vi "CRYUnflatten Graph Property.vi"(10 "Cluster Name":string, 11 "Flatten Graph Property":string) -> (0 "Error?":bool=TRUE, 2 "Flatten Graph Property Out":string, 3 "Header info":T1={"Data type"="Data            ", "Version"=1, "Dimensions"=0})   [LabVIEW 2013]
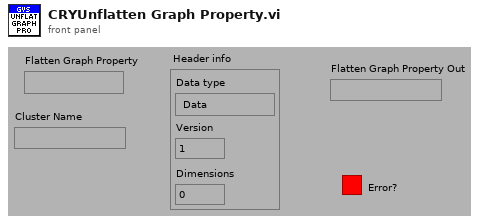
[diagram p1: front panel]
types:
  T1 = cluster{"Data type":string, "Version":u16, "Dimensions":u8}
  T2 = cluster{"unsigned byte array[0]":u8, "unsigned byte array[1]":u8, "unsigned byte array[2]":u8}
  T3 = cluster{"Image Path":string, "Show vertical scroll bar":bool, "Show horizontal scroll bar":bool}
  T4 = cluster{"Show Limits":bool, "Show Yield":bool, "Pass/Fail":bool, "Notation":u16, "Digits":u16, "Precision":u16, "Hide Traling Zeros":bool, "Show vertical scroll bar":bool, "Show horizontal scroll bar":bool, "True":string, "False":string, "Font Size":u16, "Overall/Optional":u16}
  T5 = cluster{"Show Limits":bool, "Show Yield":bool, "Overall Pass/Fail":bool, "Notation":u16, "Digits":u16, "Precision":u16, "Hide Traling Zeros":bool}
  T6 = cluster{"Show Limits":bool, "Show Yield":bool, "Overall Pass/Fail":bool, "Notation":u16, "Digits":u16, "Precision":u16, "Hide Traling Zeros":bool, "Show vertical scroll bar":bool, "Show horizontal scroll bar":bool}
  T7 = cluster{"Show Limits":bool, "Show Yield":bool, "Overall Pass/Fail":bool, "Notation":u16, "Digits":u16, "Precision":u16, "Hide Traling Zeros":bool, "Show vertical scroll bar":bool, "Show horizontal scroll bar":bool, "True":string, "False":string, "Font Size":u16}
  T8 = cluster{"Reset All Columns":bool, "Transpose":bool, "Display Units":bool, "Notation":u16, "Digits":u16, "Precision":u16, "Hide Traling Zeros":bool, "Column Width":u16, "Row Header Width":u16, "Show vertical scroll bar":bool, "Show horizontal scroll bar":bool}
  T9 = cluster{"Reset All Columns":bool, "Transpose":bool, "Display Units":bool, "Notation":u16, "Digits":u16, "Precision":u16, "Hide Traling Zeros":bool, "Column Width":u16, "Row Header Width":u16}
  T10 = cluster{"Time Steps":i32, "Frequency Bins":i32, "Type":u32, "Length":i32, "Map Type":enum16{"fire", "rainbow", "grey", "inverse grey", "ice", "original"}}
  T11 = cluster{"polar attributes":cluster{"maximum":dbl, "minimum":dbl, "clip to min":bool, "log":bool, "grid color":u32, "plot color":u32, "fmt and prec":cluster{"format":enum8{"Decimal", "Scientific", "Engineering", "Binary", "Octal", "Hex"}, "precision":u8}, "visible section":u16}, "Auto/Manual":u16, "Zero Adjust (deg)":i32, "Angle Increment (deg)":i32, "Mirror":bool, "Auto Increment":bool, "Total Rotatin (deg)":i32, "Discrete/Rannge":u16, "Show Name":bool, "CurValues":dbl[], "CurIndex":u16, "CurColors":u32[], "CurColors_Range":u32[], "CurValues_Range":dbl[], "Pen":cluster{"Width":u16, "Style":enum32{"Solid", "Dash", "Dot", "DashDot", "DashDotDot"}}, "BackgroundColor":u32}
  T12 = cluster{"polar attributes":cluster{"maximum":dbl, "minimum":dbl, "clip to min":bool, "log":bool, "grid color":u32, "plot color":u32, "fmt and prec":cluster{"format":enum8{"Decimal", "Scientific", "Engineering", "Binary", "Octal", "Hex"}, "precision":u8}, "visible section":u16}, "Auto/Manual":u16, "Zero Adjust (deg)":i32, "Angle Increment (deg)":i32, "Mirror":bool, "Auto Increment":bool, "Total Rotatin (deg)":i32, "Discrete/Rannge":u16, "Show Name":bool, "CurValues":dbl[], "CurIndex":u16, "CurColors":u32[], "CurColors_Range":u32[], "CurValues_Range":dbl[], "Pen":cluster{"Width":u16, "Style":enum32{"Solid", "Dash", "Dot", "DashDot", "DashDotDot"}}}
  T13 = cluster{"maximum":dbl, "minimum":dbl, "clip to min":bool, "log":bool, "grid color":u32, "plot color":u32, "fmt and prec":cluster{"format":enum8{"Decimal", "Scientific", "Engineering", "Binary", "Octal", "Hex"}, "precision":u8}, "visible section":u16}
  T14 = cluster{"Width":u16, "Style":enum32{"Solid", "Dash", "Dot", "DashDot", "DashDotDot"}}
  T15 = cluster{"Size":u32, "Bold":bool, "Italic":bool, "Underline":bool, "Strikethrough":bool, "Color":u32, "Font":string, "String":string, "Show vertical scroll bar":bool, "Show horizontal scroll bar":bool}
  T16 = cluster{"Size":u32, "Bold":bool, "Italic":bool, "Underline":bool, "Strikethrough":bool, "Color":u32, "Font":string, "String":string}
  T17 = cluster{"substring":string, u16, "unsigned byte array[2]":u8}
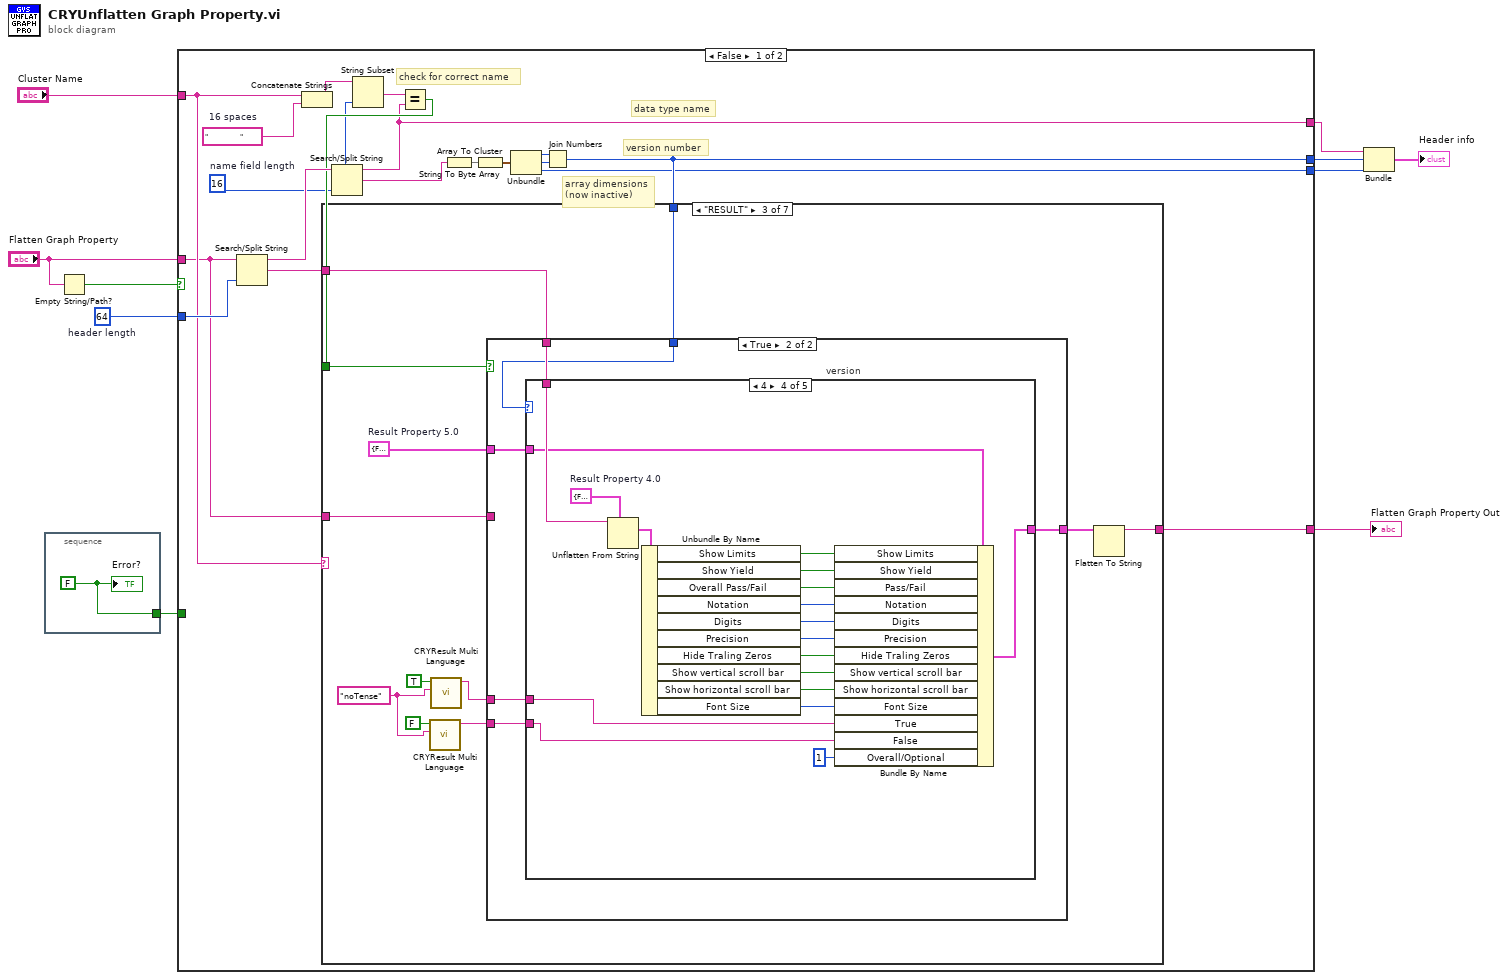
[diagram p0: block diagram]
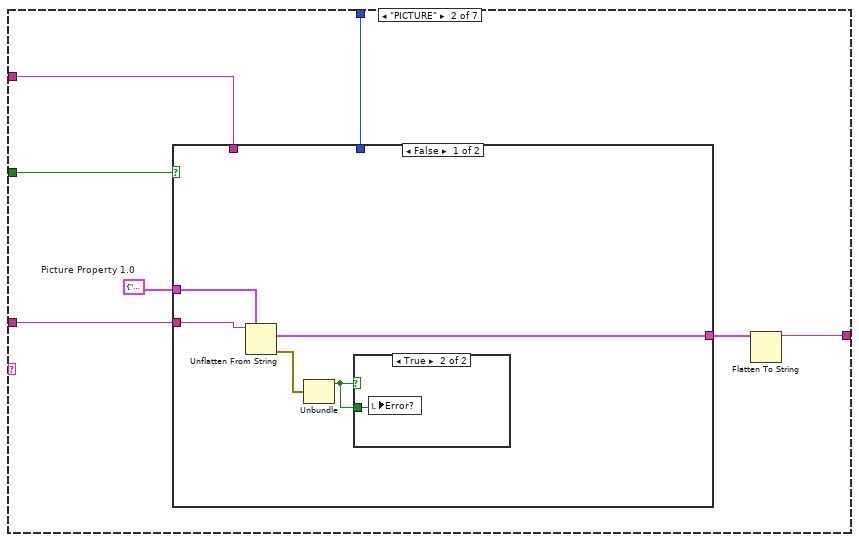
[diagram p3: hidden frame]
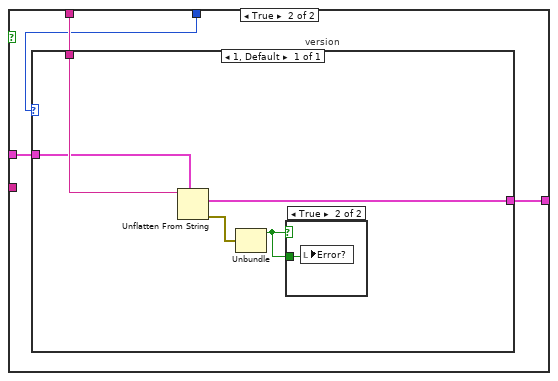
[diagram p5: hidden frame]
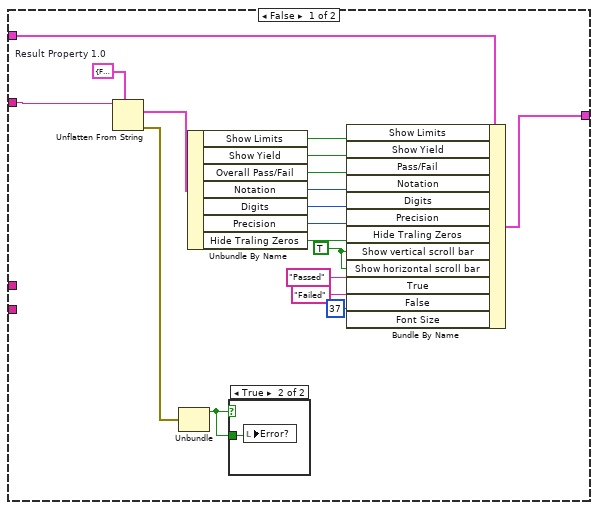
[diagram p7: hidden frame]
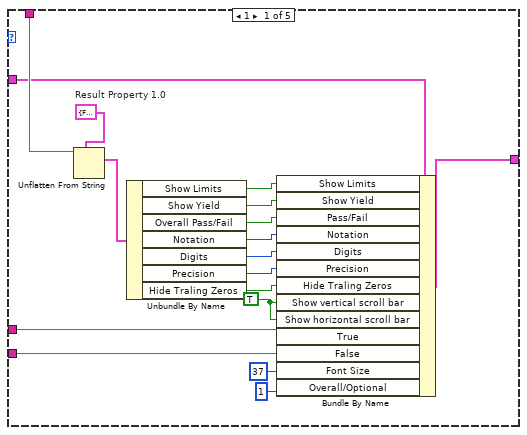
[diagram p9: hidden frame]
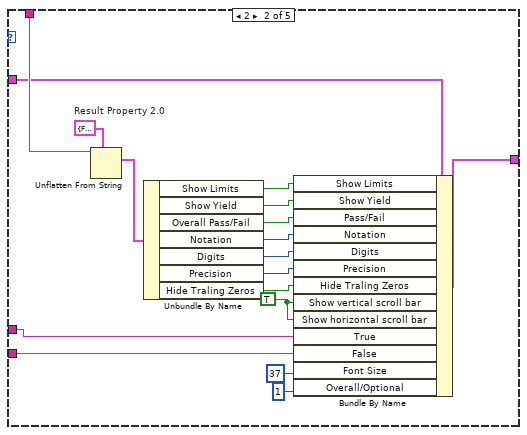
[diagram p10: hidden frame]
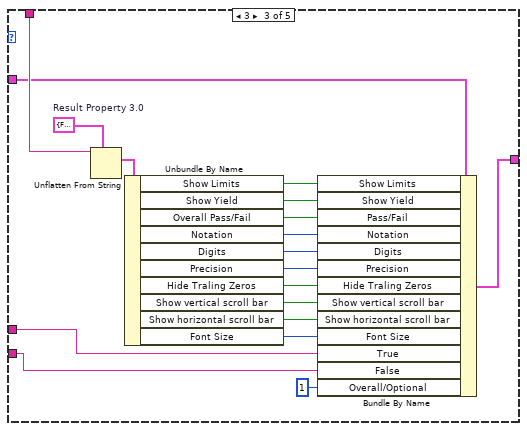
[diagram p11: hidden frame]
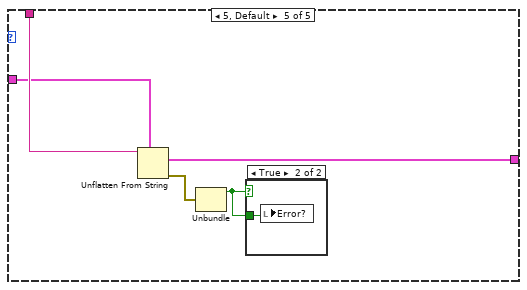
[diagram p12: hidden frame]
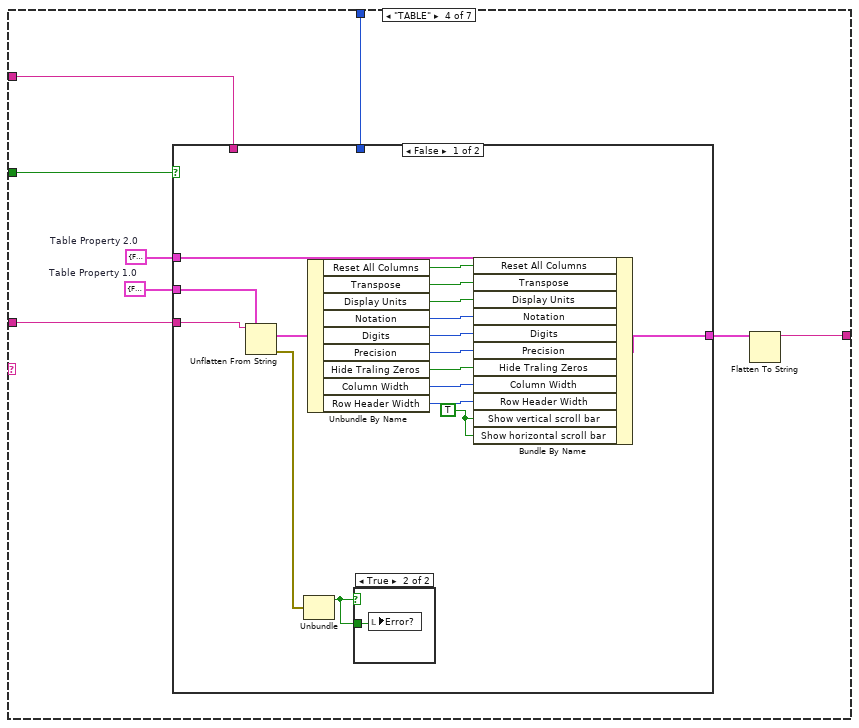
[diagram p14: hidden frame]
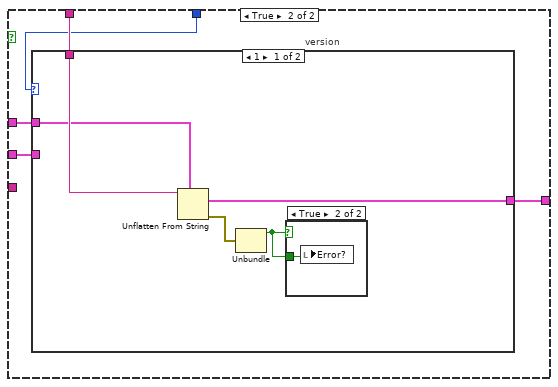
[diagram p16: hidden frame]
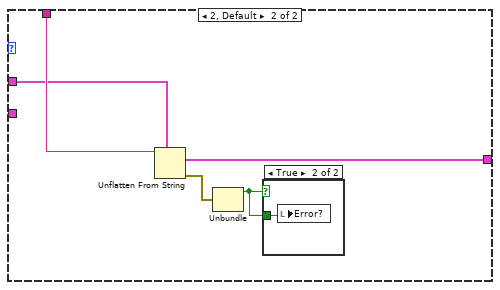
[diagram p18: hidden frame]
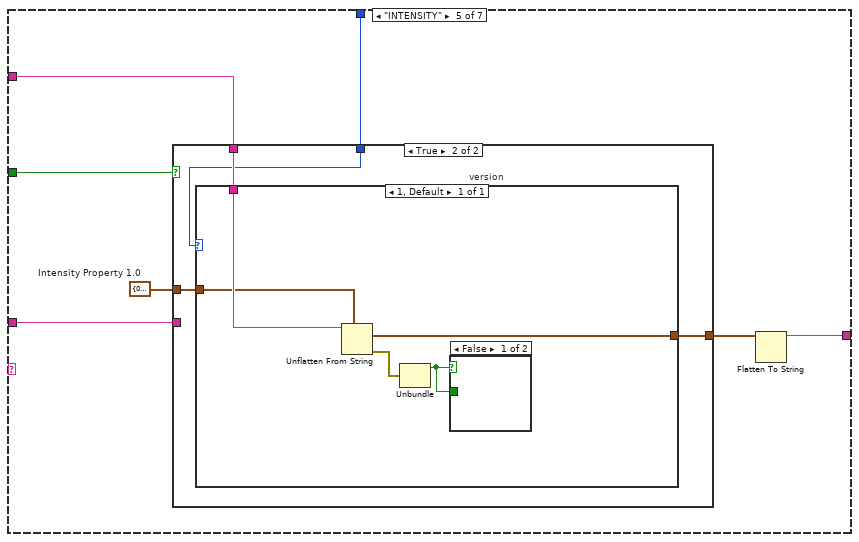
[diagram p20: hidden frame]
diagram:
  w8 = 64  # header length
  n1 = stacked-sequence {
    tunnel: [w11] -> w3
    frame #0 {
      w11 = FALSE
      "Error?" <- w11
    }
  }
  n2 = Empty String/Path?(string/path="Flatten Graph Property") -> (empty?=w9:bool)
  n3 = case shown="False" w9 {
    tunnel: "Flatten Graph Property" -> [w12 _]
    tunnel: w8 -> [w25 _]
    tunnel: [w22 u16 0] -> w6
    tunnel: [w15 u8 0] -> w7
    tunnel: [w16 "(no data input)" ("substring")] -> w5
    tunnel: w3 -> [_ _]
    tunnel: "Cluster Name" -> [w14 _]
    tunnel: [w13 "" ("data string")] -> w1
    frame False {
      w20 = "                "  # 16 spaces
      w18 = 16  # name field length
      # "check for correct name"
      # "array dimensions\n(now inactive)"
      # "version number"
      # "data type name"
      n4 = Search/Split String(string=w12, offset (0)=w25) -> (substring before match=w24:string, match + rest of string=w26:string)  [unwired: 2 out]
      n5 = Concatenate Strings(w14, w20) -> (w19:string)
      n6 = Search/Split String(string=w24, offset (0)=w18) -> (substring before match=w16:string, match + rest of string=w21:string)  [unwired: 2 out]
      n7 = String Subset(string=w19, length (rest)=w18) -> (substring=w17:string)  [unwired: 1 out]
      n8 = Equal?(x=w17, y=w16) -> (x = y?=w23:bool)
      n9 = String To Byte Array(string=w21) -> (unsigned byte array=w30:u8[])
      n10 = Array To Cluster(array=w30) -> (cluster=w29:T2)
      n11 = Unbundle(w29) -> ("unsigned byte array[0]"=w28:u8, "unsigned byte array[1]"=w27:u8, "unsigned byte array[2]"=w15:u8)
      n12 = Join Numbers(hi=w28, lo=w27) -> ((hi.lo)=w22:u16)
      n13 = case shown="\"RESULT\"" w14 {
        tunnel: w26 -> [_ w38 w66 w175 w217 w242 w322]
        tunnel: w23 -> [_ w37 w65 w174 w216 w241 w321]
        tunnel: w22 -> [_ w36 w64 w173 w215 w240 w320]
        tunnel: [w31 w33 w62 w169 w212 w237 w317] -> w13
        tunnel: w12 -> [w31 w32 w61 w168 w211 w236 w316]
        frame Default {
        }
        frame "PICTURE" {
          w35 = T3 {"Image Path"="", "Show vertical scroll bar"=FALSE, "Show horizontal scroll bar"=FALSE}  # Picture Property 1.0
          n14 = case shown="False" w37 {
            tunnel: w38 -> [_ w48]
            tunnel: w36 -> [_ w47]
            tunnel: w35 -> [w41 w46]
            tunnel: [w40 w45] -> w34
            tunnel: w32 -> [w39 _]
            frame False {
              n15 = Unflatten From String(type=w41, binary string=w39) -> (value=w40:T3, error out=w42:errorcluster)  [unwired: 1 in, 3 out]
              n16 = Unbundle(w42) -> ("status"=w43:bool)  [unwired: 2 out]
              n17 = case shown="True" w43 {
                tunnel: w43 -> [_ w44]
                frame False {
                }
                frame True {
                  n18 = local write "Error?"(w44) -> ()
                }
              }
            }
            frame True {
              n19 = case "version" shown="1, Default" w47 {
                tunnel: w48 -> [w53]
                tunnel: w46 -> [w50]
                tunnel: [w49] -> w45
                frame 1, Default {
                  n20 = Unflatten From String(type=w50, binary string=w53) -> (value=w49:T3, error out=w51:errorcluster)  [unwired: 1 in, 3 out]
                  n21 = Unbundle(w51) -> ("status"=w52:bool)  [unwired: 2 out]
                  n22 = case shown="True" w52 {
                    tunnel: w52 -> [_ w54]
                    frame False {
                    }
                    frame True {
                      n23 = local write "Error?"(w54) -> ()
                    }
                  }
                }
              }
            }
          }
          n24 = Flatten To String(anything=w34) -> (data string=w33:string)  [unwired: 3 in, 2 out]
        }
        frame "RESULT" {
          w55 = "noTense" ("sOption")
          w56 = T4 {"Show Limits"=FALSE, "Show Yield"=FALSE, "Pass/Fail"=FALSE, "Notation"=0, "Digits"=0, "Precision"=0, "Hide Traling Zeros"=FALSE, "Show vertical scroll bar"=FALSE, "Show horizontal scroll bar"=FALSE, "True"="NO ELECTRICAL SIGNAL DETECTED!\nCheck wiring and connections.", "False"="NO ELECTRICAL SIGNAL DETECTED!\nCheck wiring and connections.", "Font Size"=0, "Overall/Optional"=0}  # Result Property 5.0
          n25 = call "CRYResult Multi Language.vi"("sOption"=w55, "Verdict"=FALSE) -> ("ASCII out"=w57:string)  [unwired: 9 in]
          n26 = call "CRYResult Multi Language.vi"("sOption"=w55, "Verdict"=TRUE) -> ("ASCII out"=w58:string)  [unwired: 9 in]
          n27 = case shown="True" w65 {
            tunnel: w66 -> [_ w91]
            tunnel: w64 -> [_ w90]
            tunnel: [w71 w89] -> w63
            tunnel: w61 -> [w82 _]
            tunnel: w56 -> [w81 w88]
            tunnel: w58 -> [_ w87]
            tunnel: w57 -> [_ w86]
            frame False {
              w70 = T5 {"Show Limits"=FALSE, "Show Yield"=FALSE, "Overall Pass/Fail"=FALSE, "Notation"=0, "Digits"=0, "Precision"=0, "Hide Traling Zeros"=FALSE}  # Result Property 1.0
              w73 = TRUE ("Show vertical scroll bar")
              n28 = Unflatten From String(type=w70, binary string=w82) -> (value=w72:T5, error out=w83:errorcluster)  [unwired: 1 in, 3 out]
              n29 = Unbundle(w83) -> ("status"=w84:bool)  [unwired: 2 out]
              n30 = Unbundle By Name(w72) -> ("Show Limits"=w80:bool, "Show Yield"=w79:bool, "Overall Pass/Fail"=w78:bool, "Notation"=w77:u16, "Digits"=w76:u16, "Precision"=w75:u16, "Hide Traling Zeros"=w74:bool)
              n31 = case shown="True" w84 {
                tunnel: w84 -> [_ w85]
                frame False {
                }
                frame True {
                  n32 = local write "Error?"(w85) -> ()
                }
              }
              n33 = Bundle By Name(cluster=w81, "Show Limits"=w80, "Show Yield"=w79, "Pass/Fail"=w78, "Notation"=w77, "Digits"=w76, "Precision"=w75, "Hide Traling Zeros"=w74, "Show vertical scroll bar"=w73, "Show horizontal scroll bar"=w73, "True"="Passed", "False"="Failed", "Font Size"=u16 37) -> (w71:T4)
            }
            frame True {
              n34 = case "version" shown="4" w90 {
                tunnel: w91 -> [w108 w125 w143 w161 w166]
                tunnel: [w97 w114 w133 w151 w163] -> w89
                tunnel: w88 -> [w107 w124 w142 w160 w162]
                tunnel: w87 -> [w94 w110 w128 w147 _]
                tunnel: w86 -> [w93 w111 w127 w146 _]
                frame 1 {
                  w96 = T5 {"Show Limits"=FALSE, "Show Yield"=FALSE, "Overall Pass/Fail"=FALSE, "Notation"=0, "Digits"=0, "Precision"=0, "Hide Traling Zeros"=FALSE}  # Result Property 1.0
                  w99 = TRUE ("Show vertical scroll bar")
                  n35 = Unflatten From String(type=w96, binary string=w108) -> (value=w98:T5)  [unwired: 1 in, 4 out]
                  n36 = Unbundle By Name(w98) -> ("Show Limits"=w106:bool, "Show Yield"=w105:bool, "Overall Pass/Fail"=w104:bool, "Notation"=w103:u16, "Digits"=w102:u16, "Precision"=w101:u16, "Hide Traling Zeros"=w100:bool)
                  n37 = Bundle By Name(cluster=w107, "Show Limits"=w106, "Show Yield"=w105, "Pass/Fail"=w104, "Notation"=w103, "Digits"=w102, "Precision"=w101, "Hide Traling Zeros"=w100, "Show vertical scroll bar"=w99, "Show horizontal scroll bar"=w99, "True"=w94, "False"=w93, "Font Size"=u16 37, "Overall/Optional"=u16 1) -> (w97:T4)
                }
                frame 2 {
                  w113 = T6 {"Show Limits"=FALSE, "Show Yield"=FALSE, "Overall Pass/Fail"=FALSE, "Notation"=0, "Digits"=0, "Precision"=0, "Hide Traling Zeros"=FALSE, "Show vertical scroll bar"=FALSE, "Show horizontal scroll bar"=FALSE}  # Result Property 2.0
                  w116 = TRUE ("Show vertical scroll bar")
                  n38 = Unflatten From String(type=w113, binary string=w125) -> (value=w115:T6)  [unwired: 1 in, 4 out]
                  n39 = Unbundle By Name(w115) -> ("Show Limits"=w123:bool, "Show Yield"=w122:bool, "Overall Pass/Fail"=w121:bool, "Notation"=w120:u16, "Digits"=w119:u16, "Precision"=w118:u16, "Hide Traling Zeros"=w117:bool)
                  n40 = Bundle By Name(cluster=w124, "Show Limits"=w123, "Show Yield"=w122, "Pass/Fail"=w121, "Notation"=w120, "Digits"=w119, "Precision"=w118, "Hide Traling Zeros"=w117, "Show vertical scroll bar"=w116, "Show horizontal scroll bar"=w116, "True"=w110, "False"=w111, "Font Size"=u16 37, "Overall/Optional"=u16 1) -> (w114:T4)
                }
                frame 3 {
                  w130 = T7 {"Show Limits"=FALSE, "Show Yield"=FALSE, "Overall Pass/Fail"=FALSE, "Notation"=0, "Digits"=0, "Precision"=0, "Hide Traling Zeros"=FALSE, "Show vertical scroll bar"=FALSE, "Show horizontal scroll bar"=FALSE, "True"="", "False"="", "Font Size"=2}  # Result Property 3.0
                  n41 = Unflatten From String(type=w130, binary string=w143) -> (value=w134:T7)  [unwired: 1 in, 4 out]
                  n42 = Unbundle By Name(w134) -> ("Show Limits"=w141:bool, "Show Yield"=w140:bool, "Overall Pass/Fail"=w139:bool, "Notation"=w138:u16, "Digits"=w137:u16, "Precision"=w136:u16, "Hide Traling Zeros"=w135:bool, "Show vertical scroll bar"=w132:bool, "Show horizontal scroll bar"=w131:bool, "Font Size"=w129:u16)
                  n43 = Bundle By Name(cluster=w142, "Show Limits"=w141, "Show Yield"=w140, "Pass/Fail"=w139, "Notation"=w138, "Digits"=w137, "Precision"=w136, "Hide Traling Zeros"=w135, "Show vertical scroll bar"=w132, "Show horizontal scroll bar"=w131, "Font Size"=w129, "True"=w128, "False"=w127, "Overall/Optional"=u16 1) -> (w133:T4)
                }
                frame 4 {
                  w145 = T7 {"Show Limits"=FALSE, "Show Yield"=FALSE, "Overall Pass/Fail"=FALSE, "Notation"=0, "Digits"=0, "Precision"=0, "Hide Traling Zeros"=FALSE, "Show vertical scroll bar"=FALSE, "Show horizontal scroll bar"=FALSE, "True"="", "False"="", "Font Size"=2}  # Result Property 4.0
                  n44 = Unflatten From String(type=w145, binary string=w161) -> (value=w152:T7)  [unwired: 1 in, 4 out]
                  n45 = Unbundle By Name(w152) -> ("Show Limits"=w159:bool, "Show Yield"=w158:bool, "Overall Pass/Fail"=w157:bool, "Notation"=w156:u16, "Digits"=w155:u16, "Precision"=w154:u16, "Hide Traling Zeros"=w153:bool, "Show vertical scroll bar"=w150:bool, "Show horizontal scroll bar"=w149:bool, "Font Size"=w148:u16)
                  n46 = Bundle By Name(cluster=w160, "Show Limits"=w159, "Show Yield"=w158, "Pass/Fail"=w157, "Notation"=w156, "Digits"=w155, "Precision"=w154, "Hide Traling Zeros"=w153, "Show vertical scroll bar"=w150, "Show horizontal scroll bar"=w149, "Font Size"=w148, "True"=w147, "False"=w146, "Overall/Optional"=u16 1) -> (w151:T4)
                }
                frame 5, Default {
                  n47 = Unflatten From String(type=w162, binary string=w166) -> (value=w163:T4, error out=w164:errorcluster)  [unwired: 1 in, 3 out]
                  n48 = Unbundle(w164) -> ("status"=w165:bool)  [unwired: 2 out]
                  n49 = case shown="True" w165 {
                    tunnel: w165 -> [_ w167]
                    frame False {
                    }
                    frame True {
                      n50 = local write "Error?"(w167) -> ()
                    }
                  }
                }
              }
            }
          }
          n51 = Flatten To String(anything=w63) -> (data string=w62:string)  [unwired: 3 in, 2 out]
        }
        frame "TABLE" {
          w171 = T8 {"Reset All Columns"=FALSE, "Transpose"=FALSE, "Display Units"=FALSE, "Notation"=0, "Digits"=0, "Precision"=0, "Hide Traling Zeros"=FALSE, "Column Width"=0, "Row Header Width"=0, "Show vertical scroll bar"=FALSE, "Show horizontal scroll bar"=FALSE}  # Table Property 2.0
          w172 = T9 {"Reset All Columns"=FALSE, "Transpose"=FALSE, "Display Units"=FALSE, "Notation"=0, "Digits"=0, "Precision"=0, "Hide Traling Zeros"=FALSE, "Column Width"=0, "Row Header Width"=0}  # Table Property 1.0
          n52 = case shown="False" w174 {
            tunnel: w175 -> [_ w198]
            tunnel: w173 -> [_ w197]
            tunnel: w172 -> [w190 w196]
            tunnel: [w187 w195] -> w170
            tunnel: w171 -> [w188 w194]
            tunnel: w168 -> [w176 _]
            frame False {
              w177 = TRUE ("Show vertical scroll bar")
              n53 = Unflatten From String(type=w190, binary string=w176) -> (value=w189:T9, error out=w191:errorcluster)  [unwired: 1 in, 3 out]
              n54 = Unbundle(w191) -> ("status"=w192:bool)  [unwired: 2 out]
              n55 = Unbundle By Name(w189) -> ("Reset All Columns"=w186:bool, "Transpose"=w185:bool, "Display Units"=w184:bool, "Notation"=w183:u16, "Digits"=w182:u16, "Precision"=w181:u16, "Hide Traling Zeros"=w180:bool, "Column Width"=w179:u16, "Row Header Width"=w178:u16)
              n56 = case shown="True" w192 {
                tunnel: w192 -> [_ w193]
                frame False {
                }
                frame True {
                  n57 = local write "Error?"(w193) -> ()
                }
              }
              n58 = Bundle By Name(cluster=w188, "Reset All Columns"=w186, "Transpose"=w185, "Display Units"=w184, "Notation"=w183, "Digits"=w182, "Precision"=w181, "Hide Traling Zeros"=w180, "Column Width"=w179, "Row Header Width"=w178, "Show vertical scroll bar"=w177, "Show horizontal scroll bar"=w177) -> (w187:T8)
            }
            frame True {
              n59 = case "version" shown="1" w197 {
                tunnel: w198 -> [w203 w209]
                tunnel: w196 -> [_ _]
                tunnel: [w200 w206] -> w195
                tunnel: w194 -> [w199 w205]
                frame 1 {
                  n60 = Unflatten From String(type=w199, binary string=w203) -> (value=w200:T8, error out=w201:errorcluster)  [unwired: 1 in, 3 out]
                  n61 = Unbundle(w201) -> ("status"=w202:bool)  [unwired: 2 out]
                  n62 = case shown="True" w202 {
                    tunnel: w202 -> [_ w204]
                    frame False {
                    }
                    frame True {
                      n63 = local write "Error?"(w204) -> ()
                    }
                  }
                }
                frame 2, Default {
                  n64 = Unflatten From String(type=w205, binary string=w209) -> (value=w206:T8, error out=w207:errorcluster)  [unwired: 1 in, 3 out]
                  n65 = Unbundle(w207) -> ("status"=w208:bool)  [unwired: 2 out]
                  n66 = case shown="True" w208 {
                    tunnel: w208 -> [_ w210]
                    frame False {
                    }
                    frame True {
                      n67 = local write "Error?"(w210) -> ()
                    }
                  }
                }
              }
            }
          }
          n68 = Flatten To String(anything=w170) -> (data string=w169:string)  [unwired: 3 in, 2 out]
        }
        frame "INTENSITY" {
          w214 = T10 {"Time Steps"=0, "Frequency Bins"=0, "Type"=0, "Length"=0, "Map Type"=enum."fire"}  # Intensity Property 1.0
          n69 = case shown="True" w216 {
            tunnel: w217 -> [_ w227]
            tunnel: w215 -> [_ w226]
            tunnel: w214 -> [w220 w225]
            tunnel: [w219 w224] -> w213
            tunnel: w211 -> [w218 _]
            frame False {
              n70 = Unflatten From String(type=w220, binary string=w218) -> (value=w219:T10, error out=w221:errorcluster)  [unwired: 1 in, 3 out]
              n71 = Unbundle(w221) -> ("status"=w222:bool)  [unwired: 2 out]
              n72 = case shown="True" w222 {
                tunnel: w222 -> [_ w223]
                frame False {
                }
                frame True {
                  n73 = local write "Error?"(w223) -> ()
                }
              }
            }
            frame True {
              n74 = case "version" shown="1, Default" w226 {
                tunnel: w227 -> [w232]
                tunnel: w225 -> [w229]
                tunnel: [w228] -> w224
                frame 1, Default {
                  n75 = Unflatten From String(type=w229, binary string=w232) -> (value=w228:T10, error out=w230:errorcluster)  [unwired: 1 in, 3 out]
                  n76 = Unbundle(w230) -> ("status"=w231:bool)  [unwired: 2 out]
                  n77 = case shown="False" w231 {
                    tunnel: w231 -> [_ w233]
                    frame False {
                    }
                    frame True {
                      n78 = local write "Error?"(w233) -> ()
                    }
                  }
                }
              }
            }
          }
          n79 = Flatten To String(anything=w213) -> (data string=w212:string)  [unwired: 3 in, 2 out]
        }
        frame "POLAR" {
          w234 = T11 {"polar attributes"={"maximum"=2.0, "minimum"=0.0, "clip to min"=FALSE, "log"=FALSE, "grid color"=3381657, "plot color"=16711680, "fmt and prec"={"format"=enum."Decimal", "precision"=2}, "visible section"=4}, "Auto/Manual"=0, "Zero Adjust (deg)"=0, "Angle Increment (deg)"=0, "Mirror"=FALSE, "Auto Increment"=FALSE, "Total Rotatin (deg)"=0, "Discrete/Rannge"=0, "Show Name"=FALSE, "CurValues"=[], "CurIndex"=0, "CurColors"=[], "CurColors_Range"=[], "CurValues_Range"=[], "Pen"={"Width"=1, "Style"=enum."Solid"}, "BackgroundColor"=0}  # Polar Property 3.0
          w235 = T12 {"polar attributes"={"maximum"=2.0, "minimum"=0.0, "clip to min"=FALSE, "log"=FALSE, "grid color"=3381657, "plot color"=16711680, "fmt and prec"={"format"=enum."Decimal", "precision"=2}, "visible section"=4}, "Auto/Manual"=0, "Zero Adjust (deg)"=0, "Angle Increment (deg)"=0, "Mirror"=FALSE, "Auto Increment"=FALSE, "Total Rotatin (deg)"=0, "Discrete/Rannge"=0, "Show Name"=FALSE, "CurValues"=[], "CurIndex"=0, "CurColors"=[], "CurColors_Range"=[], "CurValues_Range"=[], "Pen"={"Width"=1, "Style"=enum."Solid"}}  # Polar Property 2.0
          w239 = T12 {"polar attributes"={"maximum"=2.0, "minimum"=0.0, "clip to min"=FALSE, "log"=FALSE, "grid color"=3381657, "plot color"=16711680, "fmt and prec"={"format"=enum."Decimal", "precision"=2}, "visible section"=4}, "Auto/Manual"=0, "Zero Adjust (deg)"=0, "Angle Increment (deg)"=0, "Mirror"=FALSE, "Auto Increment"=FALSE, "Total Rotatin (deg)"=0, "Discrete/Rannge"=0, "Show Name"=FALSE, "CurValues"=[], "CurIndex"=0, "CurColors"=[], "CurColors_Range"=[], "CurValues_Range"=[], "Pen"={"Width"=1, "Style"=enum."Solid"}}  # Polar Property 1.0
          n80 = case shown="True" w241 {
            tunnel: w242 -> [_ w269]
            tunnel: w240 -> [_ w268]
            tunnel: w239 -> [w262 w267]
            tunnel: [w245 w266] -> w238
            tunnel: w236 -> [w263 _]
            tunnel: w235 -> [_ w265]
            tunnel: w234 -> [w244 w264]
            frame False {
              n81 = Unflatten From String(type=w262, binary string=w263) -> (value=w246:T12)  [unwired: 1 in, 4 out]
              n82 = Unbundle By Name(w246) -> ("polar attributes"=w261:T13, "Auto/Manual"=w260:u16, "Zero Adjust (deg)"=w259:i32, "Angle Increment (deg)"=w258:i32, "Mirror"=w257:bool, "Auto Increment"=w256:bool, "Total Rotatin (deg)"=w255:i32, "Discrete/Rannge"=w254:u16, "Show Name"=w253:bool, "CurValues"=w252:dbl[], "CurIndex"=w251:u16, "CurColors"=w250:u32[], "CurColors_Range"=w249:u32[], "CurValues_Range"=w248:dbl[], "Pen"=w247:T14)
              n83 = Bundle By Name(cluster=w244, "polar attributes"=w261, "Auto/Manual"=w260, "Zero Adjust (deg)"=w259, "Angle Increment (deg)"=w258, "Mirror"=w257, "Auto Increment"=w256, "Total Rotatin (deg)"=w255, "Discrete/Rannge"=w254, "Show Name"=w253, "CurValues"=w252, "CurIndex"=w251, "CurColors"=w250, "CurColors_Range"=w249, "CurValues_Range"=w248, "Pen"=w247, "BackgroundColor"=u32 0) -> (w245:T11)
            }
            frame True {
              n84 = case "version" shown="3, Default" w268 {
                tunnel: w269 -> [w290 w311 w314]
                tunnel: w267 -> [w289 _ _]
                tunnel: [w287 w309 w313] -> w266
                tunnel: w265 -> [_ w291 _]
                tunnel: w264 -> [w271 w293 w312]
                frame 1 {
                  n85 = Unflatten From String(type=w289, binary string=w290) -> (value=w288:T12)  [unwired: 1 in, 4 out]
                  n86 = Unbundle By Name(w288) -> ("polar attributes"=w286:T13, "Auto/Manual"=w285:u16, "Zero Adjust (deg)"=w284:i32, "Angle Increment (deg)"=w283:i32, "Mirror"=w282:bool, "Auto Increment"=w281:bool, "Total Rotatin (deg)"=w280:i32, "Discrete/Rannge"=w279:u16, "Show Name"=w278:bool, "CurValues"=w277:dbl[], "CurIndex"=w276:u16, "CurColors"=w275:u32[], "CurColors_Range"=w274:u32[], "CurValues_Range"=w273:dbl[], "Pen"=w272:T14)
                  n87 = Bundle By Name(cluster=w271, "polar attributes"=w286, "Auto/Manual"=w285, "Zero Adjust (deg)"=w284, "Angle Increment (deg)"=w283, "Mirror"=w282, "Auto Increment"=w281, "Total Rotatin (deg)"=w280, "Discrete/Rannge"=w279, "Show Name"=w278, "CurValues"=w277, "CurIndex"=w276, "CurColors"=w275, "CurColors_Range"=w274, "CurValues_Range"=w273, "Pen"=w272, "BackgroundColor"=u32 0) -> (w287:T11)
                }
                frame 2 {
                  n88 = Unflatten From String(type=w291, binary string=w311) -> (value=w310:T12)  [unwired: 1 in, 4 out]
                  n89 = Unbundle By Name(w310) -> ("polar attributes"=w308:T13, "Auto/Manual"=w307:u16, "Zero Adjust (deg)"=w306:i32, "Angle Increment (deg)"=w305:i32, "Mirror"=w304:bool, "Auto Increment"=w303:bool, "Total Rotatin (deg)"=w302:i32, "Discrete/Rannge"=w301:u16, "Show Name"=w300:bool, "CurValues"=w299:dbl[], "CurIndex"=w298:u16, "CurColors"=w297:u32[], "CurColors_Range"=w296:u32[], "CurValues_Range"=w295:dbl[], "Pen"=w294:T14)
                  n90 = Bundle By Name(cluster=w293, "polar attributes"=w308, "Auto/Manual"=w307, "Zero Adjust (deg)"=w306, "Angle Increment (deg)"=w305, "Mirror"=w304, "Auto Increment"=w303, "Total Rotatin (deg)"=w302, "Discrete/Rannge"=w301, "Show Name"=w300, "CurValues"=w299, "CurIndex"=w298, "CurColors"=w297, "CurColors_Range"=w296, "CurValues_Range"=w295, "Pen"=w294, "BackgroundColor"=u32 0) -> (w309:T11)
                }
                frame 3, Default {
                  n91 = Unflatten From String(type=w312, binary string=w314) -> (value=w313:T11)  [unwired: 1 in, 4 out]
                }
              }
            }
          }
          n92 = Flatten To String(anything=w238) -> (data string=w237:string)  [unwired: 3 in, 2 out]
        }
        frame "TEXT" {
          w315 = T15 {"Size"=0, "Bold"=FALSE, "Italic"=FALSE, "Underline"=FALSE, "Strikethrough"=FALSE, "Color"=0, "Font"="", "String"="", "Show vertical scroll bar"=FALSE, "Show horizontal scroll bar"=FALSE}  # Text Format 2.0
          w319 = T16 {"Size"=0, "Bold"=FALSE, "Italic"=FALSE, "Underline"=FALSE, "Strikethrough"=FALSE, "Color"=0, "Font"="", "String"=""}  # Text Format 1.0
          n93 = case shown="True" w321 {
            tunnel: w322 -> [_ w344]
            tunnel: w320 -> [_ w343]
            tunnel: w319 -> [w336 w342]
            tunnel: [w323 w341] -> w318
            tunnel: w316 -> [w335 _]
            tunnel: w315 -> [w334 w340]
            frame False {
              w325 = TRUE ("Show vertical scroll bar")
              n94 = Unflatten From String(type=w336, binary string=w335) -> (value=w324:T16, error out=w337:errorcluster)  [unwired: 1 in, 3 out]
              n95 = Unbundle(w337) -> ("status"=w338:bool)  [unwired: 2 out]
              n96 = Unbundle By Name(w324) -> ("Size"=w333:u32, "Bold"=w332:bool, "Italic"=w331:bool, "Underline"=w330:bool, "Strikethrough"=w329:bool, "Color"=w328:u32, "Font"=w327:string, "String"=w326:string)
              n97 = case shown="True" w338 {
                tunnel: w338 -> [_ w339]
                frame False {
                }
                frame True {
                  n98 = local write "Error?"(w339) -> ()
                }
              }
              n99 = Bundle By Name(cluster=w334, "Size"=w333, "Bold"=w332, "Italic"=w331, "Underline"=w330, "Strikethrough"=w329, "Color"=w328, "Font"=w327, "String"=w326, "Show vertical scroll bar"=w325, "Show horizontal scroll bar"=w325) -> (w323:T15)
            }
            frame True {
              n100 = case "version" shown="2, Default" w343 {
                tunnel: w344 -> [w358 w361]
                tunnel: w342 -> [w357 _]
                tunnel: [w345 w359] -> w341
                tunnel: w340 -> [w356 w360]
                frame 1 {
                  w347 = TRUE ("Show vertical scroll bar")
                  n101 = Unflatten From String(type=w357, binary string=w358) -> (value=w346:T16)  [unwired: 1 in, 4 out]
                  n102 = Unbundle By Name(w346) -> ("Size"=w355:u32, "Bold"=w354:bool, "Italic"=w353:bool, "Underline"=w351:bool, "Strikethrough"=w352:bool, "Color"=w350:u32, "Font"=w349:string, "String"=w348:string)
                  n103 = Bundle By Name(cluster=w356, "Size"=w355, "Bold"=w354, "Italic"=w353, "Underline"=w351, "Strikethrough"=w352, "Color"=w350, "Font"=w349, "String"=w348, "Show vertical scroll bar"=w347, "Show horizontal scroll bar"=w347) -> (w345:T15)
                }
                frame 2, Default {
                  n104 = Unflatten From String(type=w360, binary string=w361) -> (value=w359:T15)  [unwired: 1 in, 4 out]
                }
              }
            }
          }
          n105 = Flatten To String(anything=w318) -> (data string=w317:string)  [unwired: 3 in, 2 out]
        }
      }
    }
    frame True {
      n106 = local write "Error?"(TRUE ("Error?")) -> ()
    }
  }
  "Flatten Graph Property Out" <- w1
  n107 = Bundle("substring"=w5, w6, "unsigned byte array[2]"=w7) -> (→"Header info":T17)  [unwired: 1 out]
